vi "Constants.vi"() -> ()   [LabVIEW 2018, in "CAN Gateway Shared.lvlib"]
doc: "Use this Global VI to access the GUIDs assigned to the page resources of the Custom Device."
uses:
  CAN Gateway Shared.lvlib
panel:
  in  "Tab Control":enum32{"GUIDS", "Constants", "Properties"}(tab)=enum."Properties"
  in  "Extra2":string="fb87be93-d633-44ab-a16f-8ceb9f52eae6"
  in  "Extra1":string="883cea95-c785-46d7-81c9-ec5413f17728"
  in  "Fault":string="d77d3844-b313-4a60-a202-612bd9173bad"
  in  "Data":string="f328f275-f50e-42e6-90d5-64fdf097d813"
  in  "Frame":string="89814871-4da4-4b84-995c-8bf20be295ce"
  in  "CAN Gateway":string="9abd83ef-7bcc-415b-9bcb-4cbfee6f4df8"
  in  "Database GUID":string="324b18e1-6d08-49a2-8541-607bc6c74f0b"
  in  "Database Section GUID":string="def5630b-577f-4ae9-9682-5f8ee445ee21"
  in  "CLUSTER":string="CLUSTER"
  in  "BAUDRATE":string="BAUDRATE"
  in  "DATA CHANNELS":string="DATA CHANNELS"
  in  "FAULT CHANNELS":string="FAULT CHANNELS"
  in  "FRAME DIRECTION":string="FRAME DIRECTION"
  in  "COMPILED DATA":string="COMPILED DATA"
  in  "ERROR NET_DUT":string="Error NET_DUT"
  in  "ERROR DUT_NET":string="Error DUT_NET"
  in  "ITERATION DURATION":string="ITERATION DURATION"
  in  "ENGINE SECTION":string="_ENGINE SECTION"
  in  "DLC LENGTH":string="DLC LENGTH"
  in  "DLC FAULT":string="DLC FAULT"
  in  "DISABLE FRAME":string="DISABLE FRAME"
  in  "FRAME CHANNELS":string="FRAME CHANNELS"
  in  "CRC":string="CRC"
  in  "TABLES":string="TABLES"
  in  "Tx FRAME":string="Tx FRAME "
  in  "Rx FRAME":string="Rx FRAME "
  in  "DB ALIAS":string="DB ALIAS"
  in  "ECU":string="ECU"
  in  "DUT PORT":string="DUT PORT"
  in  "NETWORK PORT":string="NETWORK PORT"
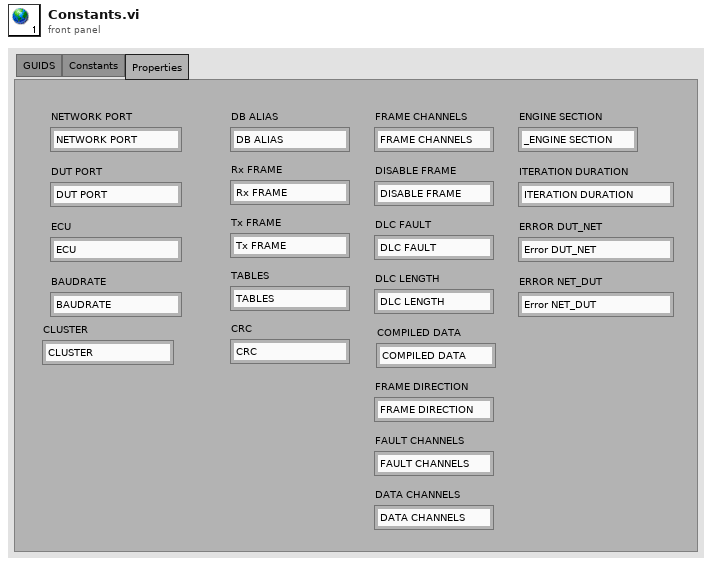
[diagram p1: front panel]
diagram:
